vi "Player Info.vi"(11 "Line Dancer in":refnum<class "Brick Wall.lvclass">) -> (0 "Defeat Speech":string, 1 "Victory Speech":string, 2 "Name":string, 3 "Line Dancer out":refnum<class "Brick Wall.lvclass">)   [LabVIEW 2015, in "Brick Wall.lvclass"]
uses:
  Brick Wall.lvclass
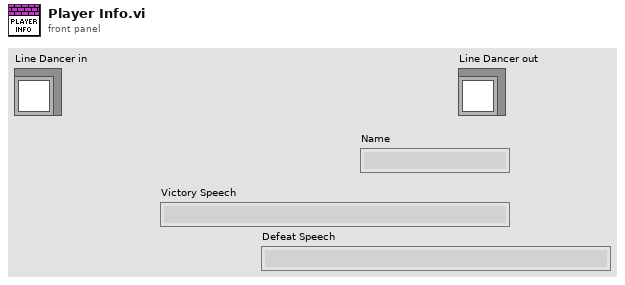
[diagram p1: front panel]
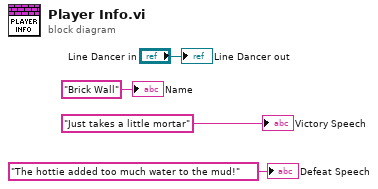
[diagram p0: block diagram]
diagram:
  "Line Dancer out" <- "Line Dancer in"
  "Name" <- "Brick Wall" ("Name")
  "Victory Speech" <- "Just takes a little mortar" ("Victory Speech")
  "Defeat Speech" <- "The hottie added too much water to the mud!" ("Defeat Speech")
